vi "PID Timing Estimation Ext.vi"(1 "R":bool, 2 "dt (s) in":dbl, 3 "Tick old":u32) -> (7 "dt (s) out":dbl, 9 "Tick":u32)   [LabVIEW 2019, in "control.lvlib"]
uses:
  control.lvlib
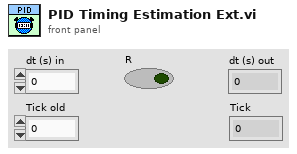
[diagram p1: front panel]
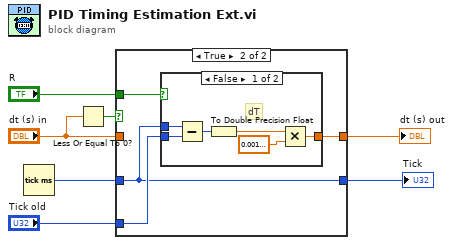
[diagram p0: block diagram]
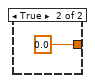
[diagram p3: hidden frame]
diagram:
  n1 = Tick Count (ms)() -> (millisecond timer value=w1:u32)
  n2 = Less Or Equal To 0?(x="dt (s) in") -> (x <= 0?=w4:bool)
  n3 = case shown="True" w4 {
    tunnel: [w9 w12] -> w6
    tunnel: "dt (s) in" -> [w9 _]
    tunnel: "R" -> [_ w13]
    tunnel: [w8 w10] -> w3
    tunnel: "Tick old" -> [_ w11]
    tunnel: w1 -> [w8 w10]
    frame False {
    }
    frame True {
      n4 = case shown="False" w13 {
        tunnel: [w14 0.0] -> w12
        tunnel: w11 -> [w18 _]
        tunnel: w10 -> [w19 _]
        frame False {
          # "dT"
          n5 = Subtract(x=w19, y=w18) -> (x-y=w15:u32)
          n6 = To Double Precision Float(number=w15) -> (double precision float=w16:dbl)
          n7 = Multiply(x=w16, y=0.0010000000474974513) -> (x*y=w14:dbl)
        }
        frame True {
        }
      }
    }
  }
  "dt (s) out" <- w6
  "Tick" <- w3
